vi "PH_Cont-601k_PSU.evt call Set Interlock Off.vi"(0 "i ref in":refnum<vi>, 2 "Instance name":string="N/A", 5 "error in":errorcluster) -> (14 "i ref out":refnum<vi>, 19 "error out":errorcluster)   [LabVIEW 2014, in "PH_Cont-601k_PSU.lvlib"]
doc: "This VI calls an event by a simple call."
uses:
  PH_Cont-601k_PSU.lvlib
  CS_Core/CSSystem/CoreLib/CoreLib.short 2 byte array.vi
  CS_Core/BaseProcess/BaseProcess.lvlib
  CS_Core/CSSystem/CoreLib/CoreLib.lvlib
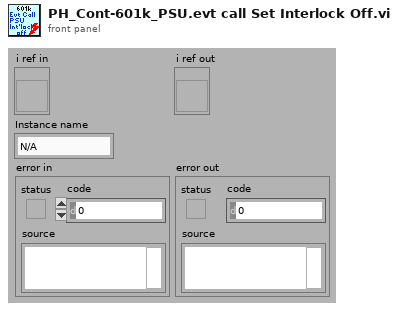
[diagram p1: front panel]
types:
  T1 = typedef "CoreDefs.rawDataType.ctl" = i8[]
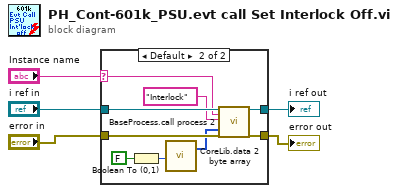
[diagram p0: block diagram]
diagram:
  n1 = case shown="Default" "Instance name" {
    selector: "Instance name" -> [_ w12]
    tunnel: [w6 w16] -> w5
    tunnel: "error in" -> [w6 w15]
    tunnel: [w7 w14] -> w3
    tunnel: "i ref in" -> [w7 w13]
    frame "", "N/A" {
    }
    frame Default {
      n2 = Boolean To (0,1)(Boolean=FALSE ("NewVal")) -> (0, 1=w10:i16)
      n3 = call-poly "CoreLib.data 2 byte array.vi"("i16"=w10) -> ("byteArray out"=w9:T1)  [unwired: 18 in]
      n4 = call "BaseProcess.call process 2.vi"("i ref in"=w13, "Object"=w12, "Selector"="Interlock", "Data"=w9, "error in (no error)"=w15) -> ("i ref out"=w14:refnum<vi>, "error out"=w16:errorcluster)  [unwired: 13 in]
    }
  }
  "error out" <- w5
  "i ref out" <- w3
